vi "Scope.vi"(0 "VISA resource name":refnum<visa-resource-name>="Scope", 1 "Gate Index":i32, 3 "Gate Length":i32=1000, 5 "Signal Channel":u16(ring)=1 format="%#_5f" items=["Channel 1", "Channel 2", "Channel 3", "Channel 4", "Math 1", "Math 2", "Math 3", "Math 4", "Reference 1", "Reference 2", "Reference 3", "Reference 4"], 9 "Trigger Channel":u16(ring) format="%#_5f" items=["Channel 1", "Channel 2", "Channel 3", "Channel 4", "Math 1", "Math 2", "Math 3", "Math 4", "Reference 1", "Reference 2", "Reference 3", "Reference 4"], 11 "Average Waveforms (10)":i32=300, 12 "Record Length (10000)":u32=10000 caption="Record Length (10000s)", 14 "Position (0.0 s)":dbl) -> (4 "Full Waveform":waveform(dbl)(graph)={"t0"=timestamp(1.815305999999491e-07 s since 1904-01-01), "dt"=5e-07, "Y"=array[10000 elements]}, 6 "Gate":dbl[](graph), 8 "Sum of Intensity (V)":dbl, 10 "Signal Arrival (ns)":dbl, 15 "Signal Duration (ns)":dbl)   [LabVIEW 2018]
uses:
  <instrlib>/Tektronix 7000 Series/Public/Configure/Configure Trigger (Edge).vi
  <instrlib>/Tektronix 7000 Series/Public/Data/Read Waveform Measurement (More).vi
  <instrlib>/Tektronix 7000 Series/Public/Data/Read (Single Waveform).vi
  <instrlib>/Tektronix 7000 Series/Tektronix 7000 Series.lvlib
panel:
  in  "Acquisition Type (0:Sample)":u16(ring)=3 items=["Sample", "Peak Detect", "Hi Res", "Average", "Envelope", "WfmDB"]
  in  "Trigger Level (0.0V)":dbl=1.0
  in  "Input Impedance (0: 1M ohm)":u16(ring)=1 items=["1M", "50"]
  in  "Vertical Range (10.0 V)":dbl=10.0
  in  "Hold for Averaging?":bool=TRUE
  out "Timebase":u32
  out "Area (V*s)":dbl
  in  "Function(0:Amplitude)":u16(ring) items=["Area", "Burst Width", "Cyc Area", "Phase"]
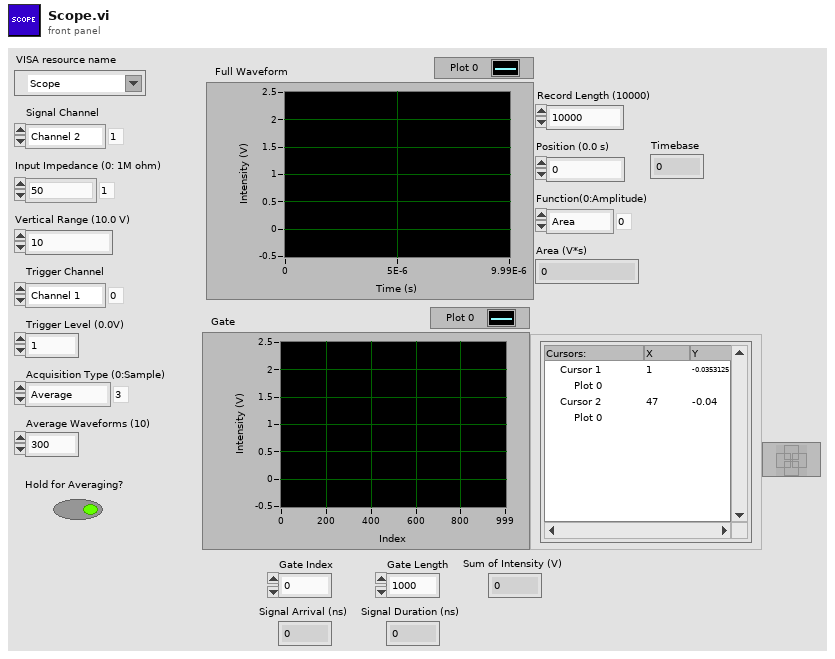
[diagram p1: front panel]
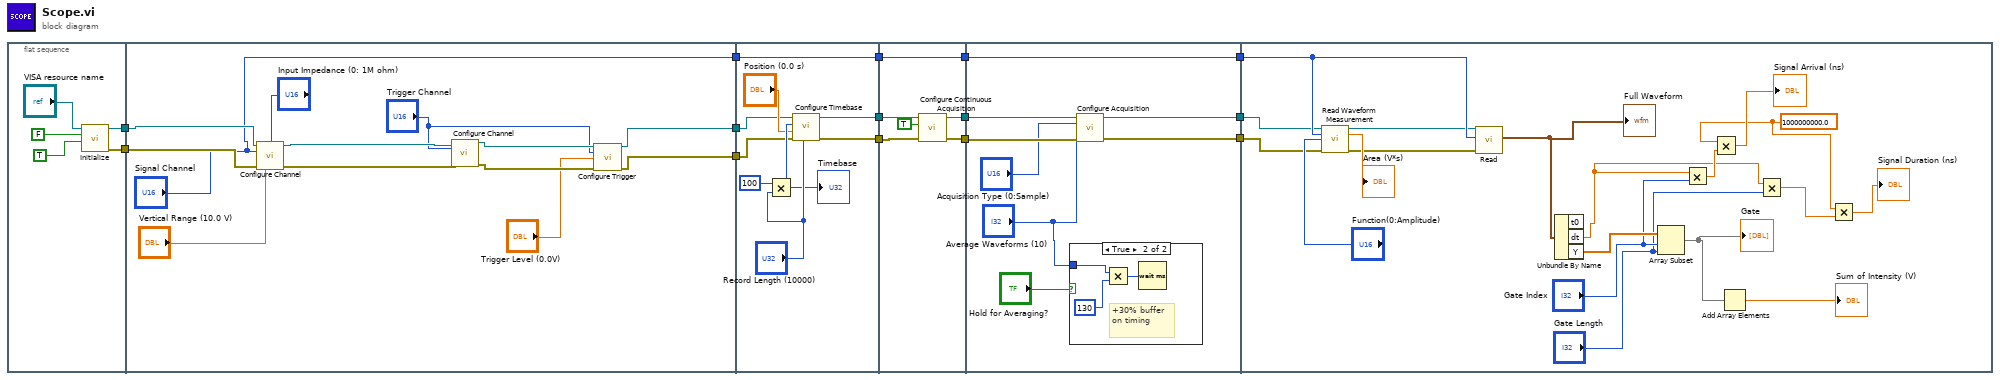
[diagram p0: block diagram]
diagram:
  n1 = flat-sequence {
    tunnel: [w18] -> w14
    tunnel: [w17] -> w13
    tunnel: w14 -> [w31]
    tunnel: w13 -> [w32]
    tunnel: ["Signal Channel"] -> w9
    tunnel: [w25] -> w2
    tunnel: [w26] -> w1
    tunnel: [w41] -> w12
    tunnel: [w40] -> w11
    tunnel: [w39] -> w10
    tunnel: w9 -> [w39]
    tunnel: w2 -> [w34]
    tunnel: w1 -> [w33]
    tunnel: [w47] -> w6
    tunnel: w10 -> [w47]
    tunnel: w11 -> [w46]
    tunnel: w12 -> [w45]
    tunnel: [w43] -> w4
    tunnel: [w42] -> w3
    tunnel: [w55] -> w8
    tunnel: [w54] -> w7
    tunnel: w6 -> [w53]
    tunnel: [w53] -> w5
    tunnel: w4 -> [w52]
    tunnel: w3 -> [w51]
    tunnel: w8 -> [w72]
    tunnel: w7 -> [w74]
    tunnel: w5 -> [w75]
    frame #0 {
      n2 = call <instrlib>:"Initialize.vi"("Reset? ( Yes)"=TRUE, "ID Query? ( Yes)"=FALSE, "VISA resource name"="VISA resource name") -> ("error out"=w17:errorcluster, "VISA resource name out"=w18:refnum<visa-resource-name>)  [unwired: 7 in]
    }
    frame #1 {
      n3 = call <instrlib>:"Configure Channel.vi"("VISA resource name"=w31, "Input Impedance (0: 1M ohm)"="Input Impedance (0: 1M ohm)", "Channel (0: Channel 1)"="Signal Channel", "error in (no error)"=w32, "Vertical Range (10.0 V)"="Vertical Range (10.0 V)") -> ("VISA resource name out"=w30:refnum<visa-resource-name>, "error out"=w29:errorcluster)  [unwired: 9 in]
      n4 = call <instrlib>:"Configure Channel.vi"("VISA resource name"=w30, "Channel (0: Channel 1)"="Trigger Channel", "error in (no error)"=w29) -> ("VISA resource name out"=w28:refnum<visa-resource-name>, "error out"=w27:errorcluster)  [unwired: 11 in]
      n5 = call-poly <instrlib>:"Configure Trigger.vi"("VISA resource name"=w28, "Source (0:Channel1)"="Trigger Channel", "Trigger Level (0.0V)"="Trigger Level (0.0V)", "error in (no error)"=w27) -> ("VISA resource name out"=w25:refnum<visa-resource-name>, "error out"=w26:errorcluster)  [unwired: 10 in]
    }
    frame #2 {
      n6 = Multiply(x=u32 100, y="Record Length (10000)") -> (x*y=w36:u32)
      "Timebase" <- w36
      n7 = call <instrlib>:"Configure Timebase.vi"("Record Length (10000)"="Record Length (10000)", "error in (no error)"=w33, "Position (0.0 s)"="Position (0.0 s)", "Timebase (4 ns)"=w36, "VISA resource name"=w34) -> ("error out"=w40:errorcluster, "VISA resource name out"=w41:refnum<visa-resource-name>)  [unwired: 5 in]
    }
    frame #3 {
      n8 = call <instrlib>:"Configure Continuous Acquisition.vi"("error in (no error)"=w46, "Enable Continuous Acquisition Mode (True)"=TRUE, "VISA resource name"=w45) -> ("error out"=w42:errorcluster, "VISA resource name out"=w43:refnum<visa-resource-name>)  [unwired: 7 in]
    }
    frame #4 {
      n9 = case shown="True" "Hold for Averaging?" {
        tunnel: "Average Waveforms (10)" -> [_ w56]
        frame False {
        }
        frame True {
          # "+30% buffer on timing"
          n10 = Multiply(x=w56, y=u32 130) -> (x*y=w58:u32)
          n11 = Wait (ms)(milliseconds to wait=w58) -> ()  [unwired: 1 out]
        }
      }
      n12 = call <instrlib>:"Configure Acquisition.vi"("VISA resource name"=w52, "Acquisition Type (0:Sample)"="Acquisition Type (0:Sample)", "Average Waveforms (10)"="Average Waveforms (10)", "error in (no error)"=w51) -> ("VISA resource name out"=w55:refnum<visa-resource-name>, "error out"=w54:errorcluster)  [unwired: 10 in]
    }
    frame #5 {
      w63 = 1000000000.0 ("x")
      n13 = call-poly <instrlib>:"Read Waveform Measurement.vi"("VISA resource name"=w72, "Channel1 (0:Channel1)"=w75, "Function(0:Amplitude)"="Function(0:Amplitude)", "error in (no error)"=w74) -> ("VISA resource name out"=w71:refnum<visa-resource-name>, "Measurement"=→"Area (V*s)":dbl, "error out"=w73:errorcluster)  [unwired: 9 in]
      n14 = call-poly <instrlib>:"Read.vi"("error in (no error)"=w73, "Channel (0: Channel 1)"=w75, "VISA resource name"=w71) -> ("Waveform Data"=w68:waveform(dbl))  [unwired: 6 in, 2 out]
      "Full Waveform" <- w68
      n15 = Unbundle By Name(w68) -> ("dt"=w60:dbl, "Y"=w67:dbl[])  [unwired: 1 out]
      n16 = Array Subset(array=w67, index="Gate Index", length="Gate Length") -> (w69:dbl[])
      "Gate" <- w69
      n17 = Multiply(x=w60, y="Gate Index") -> (x*y=w62:dbl)
      n18 = Multiply(x=w63, y=w62) -> (x*y=→"Signal Arrival (ns)":dbl)
      n19 = Add Array Elements(numeric array=w69) -> (sum=→"Sum of Intensity (V)":dbl)
      n20 = Multiply(x=w60, y="Gate Length") -> (x*y=w59:dbl)
      n21 = Multiply(x=w63, y=w59) -> (x*y=→"Signal Duration (ns)":dbl)
    }
  }
